vi "Controller and 3D Model - Bluetooth.vi"() -> ()   [LabVIEW 2012]
panel:
  in  "Axis plots":enum32{"X Axis", "Y Axis"}(tab)
  out "X Filtered":i32(graph)
  out "X Chart":i32(graph)
  out "Y Chart":i32(graph)
  out "Y Filtered":i32(graph)
  in  "Stop":bool
  in  "UART configuration and 3D Model":T1(tab)=enum."3D Model View"
  in  "Loop wait [ms]":u32
  in  "Waiting time after sent [ms]":u32
  in  "Hexadecimal Input String":string="03"
  in  "Bluetooth time limit [ms]":i32=1000
  out "Device Name":string
  in  "Sample quantity":i32=64
  in  "STL File Path":path=path "C:/Users/Marcin_2/Documents/Quadrocopter/QuadroTwins-master/QuadroController LabView/quadro-controller/Controller and 3D Model - Bluetooth/quadro.stl"
  out "3D Picture Control":refnum<vi>(3d-picture)
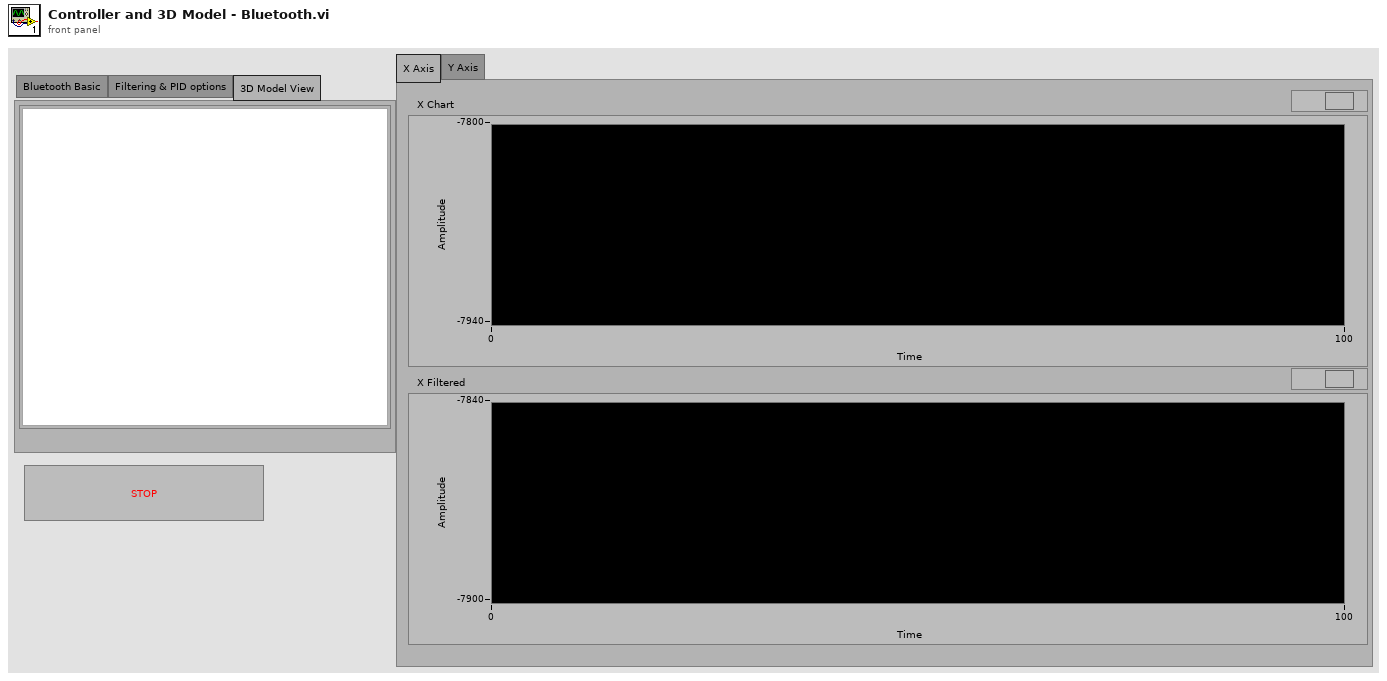
[diagram p1: front panel]
types:
  T1 = enum32{"Bluetooth Basic", "Filtering & PID options", "3D Model View"}
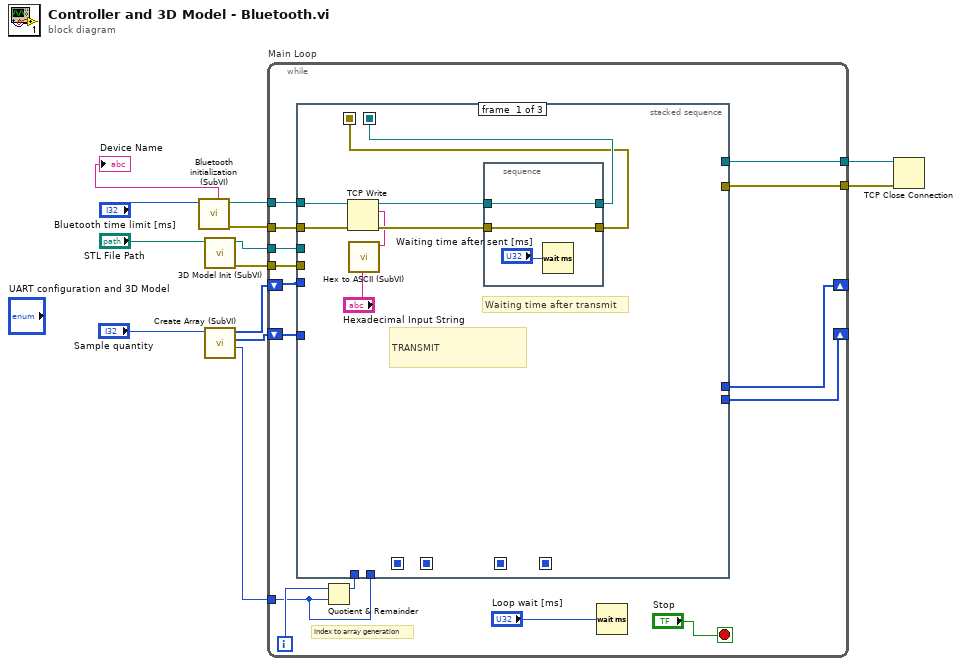
[diagram p0: block diagram]
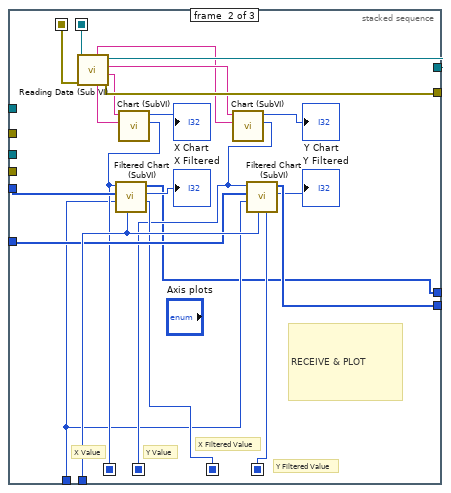
[diagram p2: hidden frame]
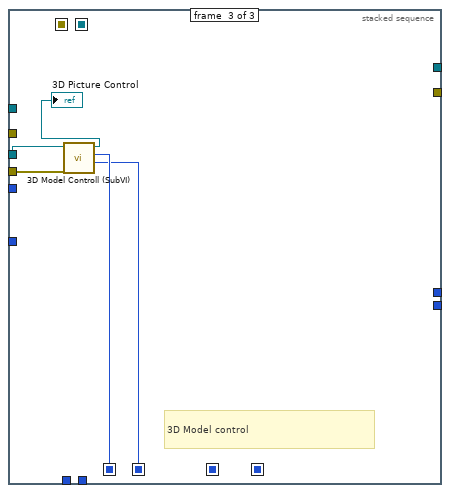
[diagram p3: hidden frame]
diagram:
  n1 = call "Bluetooth initialization (SubVI).vi"("time limit ms (10000)"="Bluetooth time limit [ms]") -> ("error out"=w7:errorcluster, "Bluetooth Network Connection out"=w11:refnum<k31>, "Device Name"=→"Device Name":string)  [unwired: 5 in, 3 out]
  n2 = call "3D Model Init (SubVI).vi"("STL File Path"="STL File Path") -> ("error out"=w13:errorcluster, "SceneObject out"=w5:refnum<vi>)  [unwired: 9 in]
  n3 = call "Create Array (SubVI).vi"("Sample quantity in"="Sample quantity") -> ("Sample quantity out"=w2:i32, "Array"=w3:i32[], "Array 2"=w12:i32[])  [unwired: 8 in]
  n4 = while "Main Loop" {
    tunnel: w11 -> [w28]
    tunnel: w7 -> [w27]
    tunnel: [w23] -> w8
    tunnel: [w24] -> w9
    tunnel: w5 -> [w22]
    tunnel: w13 -> [w21]
    shift-right: [w18] -> _
    shift-left: w12 -> [w17]
    tunnel: w2 -> [w16]
    shift-right: [w14] -> _
    shift-left: w3 -> [w15]
    i -> [w20]
    stop <- "Stop" stop-if-true
    # "Index to array generation"
    n5 = Quotient & Remainder(x=w20, y=w16) -> (x-y*floor(x/y)=w19:i32)  [unwired: 1 out]
    n6 = stacked-sequence "1 - Transmit, 2 - Receive" {
      seq-local: [w30 _ _] -> [_ w60 _]
      seq-local: [w29 _ _] -> [_ w61 _]
      seq-local: [_ w45 _] -> [_ _ w66]
      seq-local: [_ w44 _] -> [_ _ w64]
      seq-local: [_ w46 _] -> [_ _ _]
      seq-local: [_ w43 _] -> [_ _ _]
      tunnel: w28 -> [w35 _ _]
      tunnel: w27 -> [w34 _ _]
      tunnel: [_ w59 _] -> w24
      tunnel: [_ w58 _] -> w23
      tunnel: w22 -> [_ _ w65]
      tunnel: w21 -> [_ _ w62]
      tunnel: w17 -> [_ w57 _]
      tunnel: w19 -> [_ w42 _]
      tunnel: [_ w40 _] -> w18
      tunnel: w16 -> [_ w55 _]
      tunnel: w15 -> [_ w47 _]
      tunnel: [_ w56 _] -> w14
      frame #0 {
        # "TRANSMIT"
        # "Waiting time after transmit"
        n7 = call "Hex to ASCII (SubVI).vi"("Hexadecimal Input String"="Hexadecimal Input String") -> ("String"=w31:string)  [unwired: 10 in]
        n8 = TCP Write(connection ID=w35, data in=w31, error in (no error)=w34) -> (connection ID out=w32:refnum<k31>, error out=w33:errorcluster)  [unwired: 1 in, 1 out]
        n9 = stacked-sequence "Waiting time" {
          tunnel: [w38] -> w30
          tunnel: w32 -> [w38]
          tunnel: [w37] -> w29
          tunnel: w33 -> [w37]
          frame #0 {
            n10 = Wait (ms)(milliseconds to wait="Waiting time after sent [ms]") -> ()  [unwired: 1 out]
          }
        }
      }
      frame #1 {
        # "Y Filtered Value"
        # "X Filtered Value"
        # "X Value"
        # "Y Value"
        # "RECEIVE & PLOT"
        n11 = call "Reading Data (Sub VI).vi"("error in (no error)"=w61, "Bluetooth Network Connection in"=w60) -> ("error out"=w59:errorcluster, "Sign bytes X"=w54:string, "Sign bytes Y"=w50:string, "Bluetooth Network Connection out"=w58:refnum<k31>, "X data"=w53:string, "Y data"=w49:string)  [unwired: 4 in]
        n12 = call "Chart (SubVI).vi"("data"=w53, "Sign bytes"=w54) -> ("Numeric"=w45:i32, "Chart"=→"X Chart":i32)  [unwired: 8 in]
        n13 = call "Filtered Chart (SubVI).vi"("Sample quantity"=w55, "Numeric in"=w42, "Array in"=w57, "Numeric 3"=w45) -> ("Numeric out"=w46:i32, "Filtered"=→"X Filtered":i32, "Array out"=w40:i32[])  [unwired: 5 in]
        n14 = call "Chart (SubVI).vi"("data"=w49, "Sign bytes"=w50) -> ("Numeric"=w44:i32, "Chart"=→"Y Chart":i32)  [unwired: 8 in]
        n15 = call "Filtered Chart (SubVI).vi"("Sample quantity"=w55, "Numeric in"=w42, "Array in"=w47, "Numeric 3"=w44) -> ("Numeric out"=w43:i32, "Filtered"=→"Y Filtered":i32, "Array out"=w56:i32[])  [unwired: 5 in]
      }
      frame #2 {
        # "3D Model control"
        n16 = call "3D Model Controll (SubVI).vi"("error in (no error)"=w62, "Numeric"=w64, "Numeric 2"=w66, "SceneObject in"=w65) -> ("SceneNode out"=→"3D Picture Control":refnum<vi>)  [unwired: 7 in]
      }
    }
    n17 = Wait (ms)(milliseconds to wait="Loop wait [ms]") -> ()  [unwired: 1 out]
  }
  n18 = TCP Close Connection(connection ID=w8, error in (no error)=w9) -> ()  [unwired: 1 in, 2 out]
